vi "Read.Initialize.vi"(8 "error in (no error)":errorcluster, 11 "Settings":cluster{"Refs":T1[], "Values":dbl[]} {"Refs"."Data Reference" format="%.0x"}) -> (0 "error out":errorcluster, 3 "Read out":refnum<class "Read.lvclass">)   [LabVIEW 2015, in "Data Access Engine.lvlib" / "Read.lvclass"]
uses:
  Read.lvclass
  <vilib>/NI Veristand/Custom Device API/Block Data Reference.ctl
  <vilib>/NI Veristand/Custom Device API/Data Reference.ctl
  Read.lvclass/Read.ctl
  <vilib>/NI Veristand/Custom Device API/Custom Device API.lvlib
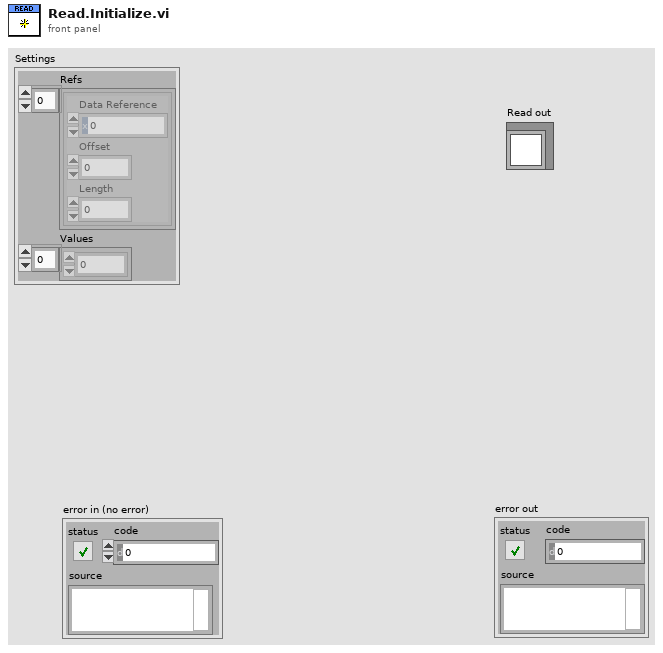
[diagram p1: front panel]
types:
  T1 = typedef "Custom Device API.lvlib/Block Data Reference.ctl" = cluster{"Data Reference":T2, "Offset":u64, "Length":u64}
  T2 = typedef "Custom Device API.lvlib/Data Reference.ctl" = i32
  T3 = cluster{"read mode":enum16{"polling", "blocking"}, "write mode":enum16{"polling", "blocking"}}
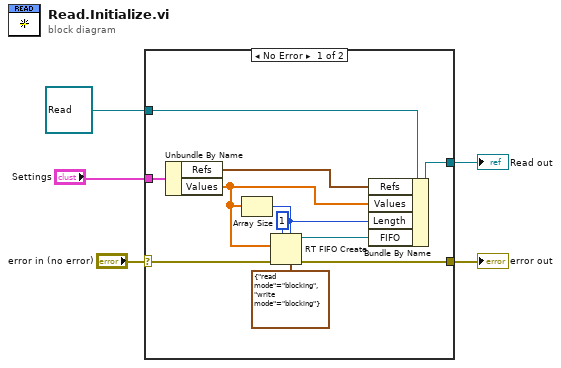
[diagram p0: block diagram]
diagram:
  n1 = case shown="No Error" "error in (no error)" {
    selector: "error in (no error)" -> [w10 w18]
    tunnel: [w14 w18] -> w5
    tunnel: "Settings" -> [w12 _]
    tunnel: [w11 w17] -> w2
    tunnel: refnum<class "Read.lvclass"> refnum ("Read out") -> [w7 w17]
    frame No Error {
      n2 = Unbundle By Name(w12) -> ("Refs"=w9:T1[], "Values"=w8:dbl[])
      n3 = Array Size(array=w8) -> (size(s)=w6:i32)
      n4 = RT FIFO Create(1:w8, 3:w10, 4:u32 1 ("size (10)"), 6:w6, 7:T3 {"read mode"=enum."blocking", "write mode"=enum."blocking"} ("r/w modes (polling,polling)")) -> (8:w16:refnum<k33>, 11:w14:errorcluster)  [unwired: 3 in, 1 out]
      n5 = Bundle By Name(cluster=w7, "Refs"=w9, "Values"=w8, "Length"=w6, "FIFO"=w16) -> (w11:refnum<class "Read.lvclass">)
    }
    frame Error {
    }
  }
  "error out" <- w5
  "Read out" <- w2
